vi "Power Line Monitor.vi"() -> ()   [LabVIEW 2023]
doc: "This example shows the application of autoregressive (AR) modeling in monitoring the condition of a power line.\n\nIn normal condition, a power signal from a grid is a stationary time series. If you build an AR model for the stationary time series, the modeling errors are small. However, if the power grid is not working properly due to variant loads or failure, the signal becomes a nonstationary time series. If you build an AR model for the nonstationary time series, the modeling errors increase. \n\nThis example builds an AR model for a signal from the power grid using the TSA AR Modeling VI. \n\n<b>Instructions:</b>\nRun this VI. Observe when the fault occurs."
uses:
  <vilib>/addons/Time Series Analysis/Utilities.llb/TSA Data.ctl
  <vilib>/addons/Time Series Analysis/Modeling and Prediction.llb/TSA AR Modeling (Array).vi
  <vilib>/addons/Time Series Analysis/Statistical Analysis.llb/TSA Deviation and Variance (Array).vi
  <vilib>/addons/_Advanced Signal Processing/NI_AdvSigProcTSA.lvlib
panel:
  out "Main AR Coefficient":dbl(graph)
  in  "stop":bool
  in  "Threshold":dbl(slide)=48.9795918367347 scale=0.0..100.0
  out "Fault?":bool
  out "Noise Variance":cluster{"variance":dbl, "Threshold":dbl}(graph)
  out "Power Line Time Series":dbl(graph)
  # "Overview: Shows the application of autoregressive (AR) modeling in monitoring the condition of a power line.\nRequirements: LabVIEW Full Development System, Advanced Signal Processing Toolkit\nInstructions: \n1. Run this VI. Observe when the fault occurs.\n2. Click Stop to stop the VI."
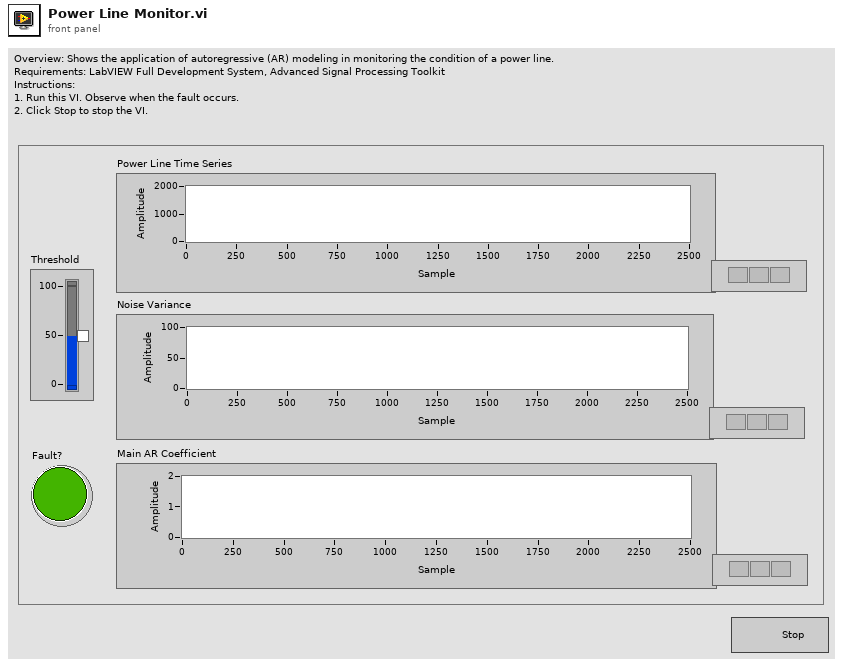
[diagram p1: front panel]
types:
  T1 = typedef "NI_AdvSigProcTSA.lvlib/TSA Data.ctl" = u16
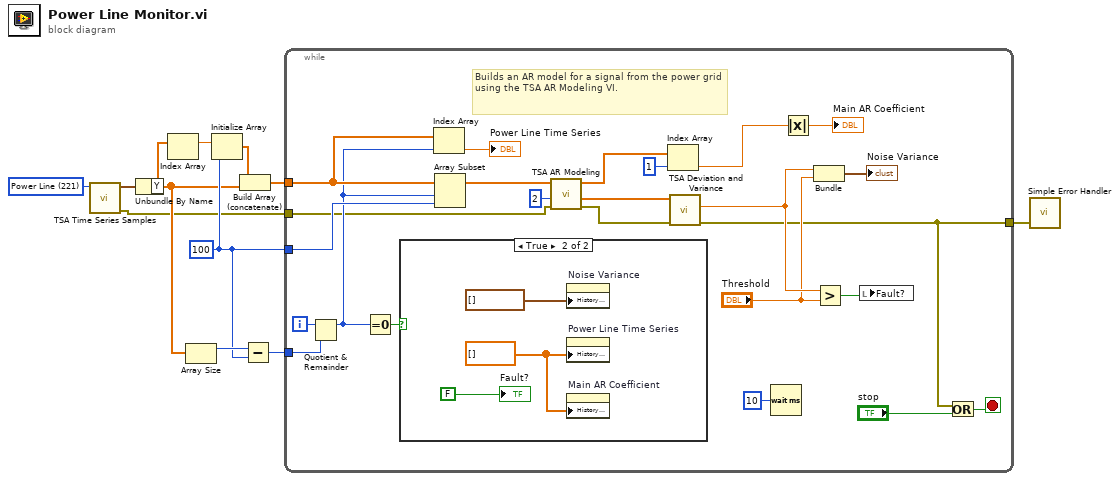
[diagram p0: block diagram]
diagram:
  w3 = T1 221 items=["Kobe Earthquake"=201, "EEG"=210, "Bearing Vibration (simulated)"=211, "Period Product Sales"=214, "Beam Vibration (nonlinear)"=217, "Beam Vibration (linear)"=218, "Signal With Echo"=219, "Engine Knocking"=220, "Power Line"=221, "-"=200, "Beam Deflections (multivariate)"=207, "Structure Vibration (multivariate)"=208, "Human MEG (multivariate)"=222] ("data")
  w6 = 100
  n1 = call <vilib>:"TSA Time Series Samples.vi"("data"=w3) -> ("error out"=w1:errorcluster, "univariate time series"=w5:waveform(dbl))  [unwired: 1 in, 8 out]
  n2 = Unbundle By Name(w5) -> ("Y"=w4:dbl[])
  n3 = Index Array(array=w4) -> (element=w9:dbl)  [unwired: 1 in]
  n4 = Array Size(array=w4) -> (size(s)=w7:i32)
  n5 = Initialize Array(w9, w6) -> (w10:dbl[])
  n6 = Build Array (concatenate)(w10, w4) -> (w11:dbl[])
  n7 = Subtract(x=w7, y=w6) -> (x-y=w8:i32)
  n8 = while {
    tunnel: w11 -> [w31]
    tunnel: w6 -> [w34]
    tunnel: w8 -> [w28]
    tunnel: [w13] -> w2
    tunnel: w1 -> [w12]
    i -> [w27]
    stop <- w14 stop-if-true
    # "Builds an AR model for a signal from the power grid using the TSA AR Modeling VI."
    n9 = Quotient & Remainder(x=w27, y=w28) -> (x-y*floor(x/y)=w26:i32)  [unwired: 1 out]
    n10 = Equal To 0?(x=w26) -> (x = 0?=w29:bool)
    n11 = case shown="True" w29 {
      frame False {
      }
      frame True {
        w38 = dbl[] [] ("History Data")
        n12 = property on="Noise Variance" class="WFChart (strict)"("History Data"=cluster{"variance":dbl, "Threshold":dbl}[] []) -> ()  [unwired: 2 in, 2 out]
        n13 = property on="Power Line Time Series" class="WFChart (strict)"("History Data"=w38) -> ()  [unwired: 2 in, 2 out]
        n14 = property on="Main AR Coefficient" class="WFChart (strict)"("History Data"=w38) -> ()  [unwired: 2 in, 2 out]
        "Fault?" <- FALSE ("Fault?")
      }
    }
    n15 = Index Array(array=w31, index=w26) -> (element=→"Power Line Time Series":dbl)
    n16 = Array Subset(array=w31, index=w26, length=w34) -> (w25:dbl[])
    n17 = call-poly <vilib>:"TSA AR Modeling.vi"("error in (no error)"=w12, "AR order"=2, "Xt"=w25) -> ("error out"=w15:errorcluster, "noise"=w22:dbl[], "AR coefficients"=w24:dbl[])  [unwired: 1 in, 5 out]
    n18 = Index Array(array=w24, index=1) -> (element=w23:dbl)
    n19 = call-poly <vilib>:"TSA Deviation and Variance.vi"("error in (no error)"=w15, "Xt"=w22) -> ("error out"=w13:errorcluster, "variance"=w21:dbl)  [unwired: 1 in, 7 out]
    n20 = Wait (ms)(milliseconds to wait=u32 10 ("millisecond multiple")) -> ()  [unwired: 1 out]
    n21 = Absolute Value(x=w23) -> (abs(x)=→"Main AR Coefficient":dbl)
    n22 = Bundle("variance"=w21, "Threshold"="Threshold") -> (→"Noise Variance":cluster{"variance":dbl, "Threshold":dbl})  [unwired: 1 out]
    n23 = Greater?(x=w21, y="Threshold") -> (0:w18:bool)
    n24 = local write "Fault?"(w18) -> ()
    n25 = Or(x=w13, y="stop") -> (x .or. y?=w14:bool)
  }
  n26 = call <vilib>:"Simple Error Handler.vi"("error in (no error)"=w2) -> ()  [unwired: 1 in, 8 out]
